vi "Update Core.vi"(8 "error in (no error)":errorcluster, 11 "Level Controller in":refnum<class "Timed Loop Actor.lvclass">) -> (0 "error out":errorcluster, 3 "Level Controller out":refnum<class "Timed Loop Actor.lvclass">)   [LabVIEW 2025, in "Timed Loop Actor.lvlib" / "Timed Loop Actor.lvclass"]
doc: "This VI specifies the action that a timed loop controller should take every time the loop executes. Children may put any action they want into their override VIs, but they should be aware that the action should be able to execute within the time specified in \"poll rate\". Child classes should take care to only include functionality that is deterministic -- no asynchronous functions, no operations that require the UI thread, etc. The Timed Loop Controller class is designed to provide deterministic repetitive behavior when deployed on a real-time system, and any code that isn't deterministic can cause odd system faults that are hard to debug."
uses:
  Timed Loop Actor.lvclass
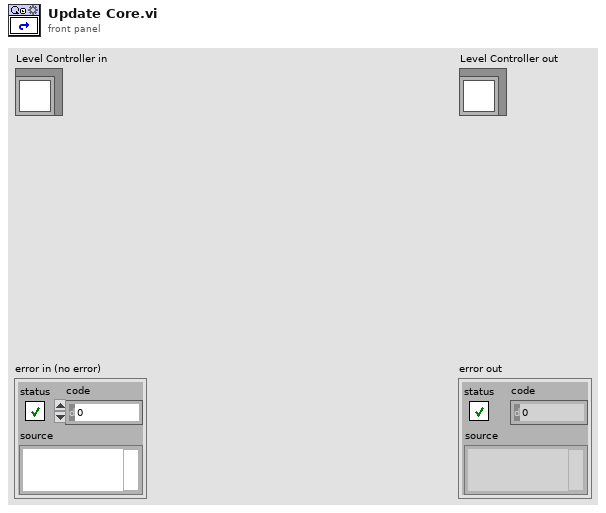
[diagram p1: front panel]
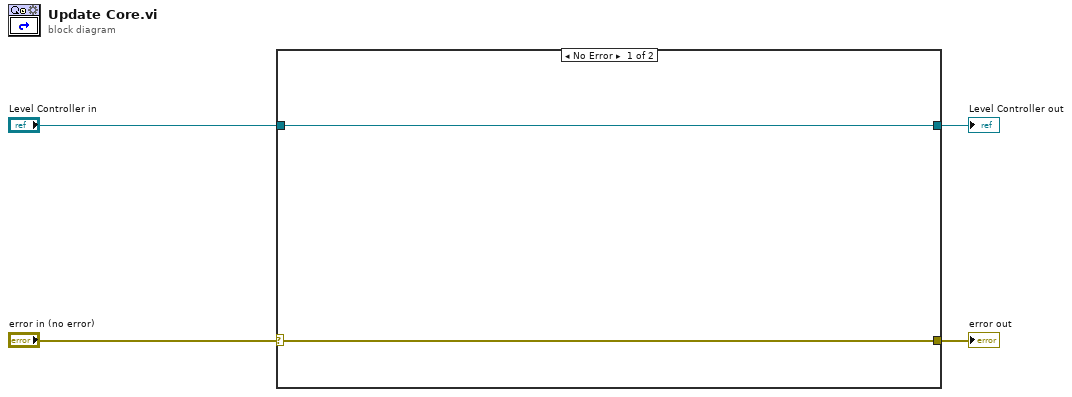
[diagram p0: block diagram]
diagram:
  n1 = case shown="No Error" "error in (no error)" {
    selector: "error in (no error)" -> [w5 w8]
    tunnel: [w5 w8] -> w3
    tunnel: [w6 w7] -> w1
    tunnel: "Level Controller in" -> [w6 w7]
    frame No Error {
    }
    frame Error {
    }
  }
  "error out" <- w3
  "Level Controller out" <- w1
